vi "DragPositionScreenToPanel.vi"(8 "error in (no error)":errorcluster, 10 "DragPosition (Screen)":i32, 11 "OrderSelection in":refnum<class "OrderSelection.lvclass">) -> (0 "error out":errorcluster, 2 "DragPosition (Panel)":i32, 3 "OrderSelection out":refnum<class "OrderSelection.lvclass">)   [LabVIEW 2020, in "OrderSelection.lvclass"]
uses:
  OrderSelection.lvclass
  C:/Program Files/National Instruments/LabVIEW 2020/vi.lib/QSI/QControls/QControl Classes/GObject/GObject.lvclass
  C:/Program Files/National Instruments/LabVIEW 2020/vi.lib/QSI/QControls/QControl Classes/Generic/Generic.lvclass
  <vilib>/Utility/miscctls.llb/LVPointTypeDef.ctl
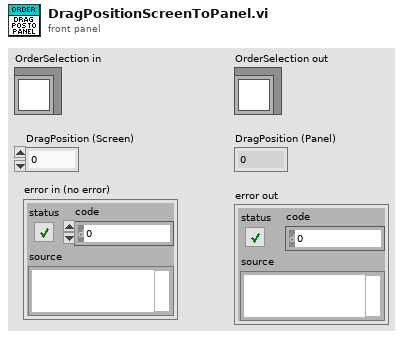
[diagram p1: front panel]
types:
  T1 = typedef "LVPointTypeDef.ctl" = cluster{"Horizontal":i16, "Vertical":i16}
  T2 = typedef "LVRectTypeDef.ctl" = cluster{"Left":i16, "Top":i16, "Right":i16, "Bottom":i16}
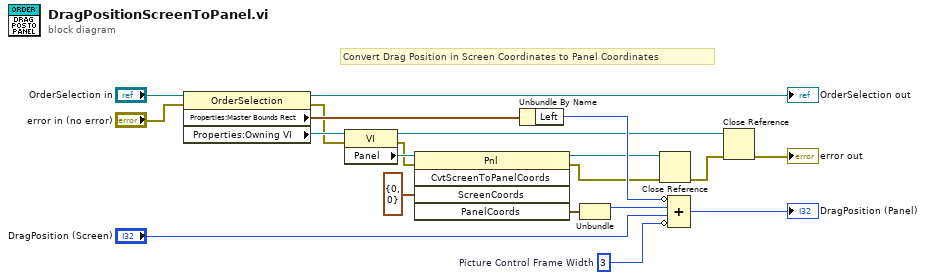
[diagram p0: block diagram]
diagram:
  w15 = 3  # Picture Control Frame Width
  # "Convert Drag Position in Screen Coordinates to Panel Coordinates"
  n1 = property class="OrderSelection"(reference="OrderSelection in", error in="error in (no error)") -> (reference out=→"OrderSelection out":refnum<class "OrderSelection.lvclass">, error out=w7:errorcluster, "Properties:Master Bounds Rect"=w14:T2, "Properties:Owning VI"=w9:refnum<vi>)
  n2 = property class="VI"(reference=w9, error in=w7) -> (reference out=w3:refnum<vi>, error out=w6:errorcluster, "Panel"=w10:refnum<vi>)
  n3 = invoke class="Pnl" method="CvtScreenToPanelCoords"(reference=w10, error in=w6, "ScreenCoords"=T1 {"Horizontal"=0, "Vertical"=0} ("Screen Coordinates")) -> (reference out=w4:refnum<vi>, error out=w5:errorcluster, "PanelCoords"=w12:T1)  [unwired: 2 in, 2 out]
  n4 = Unbundle By Name(w14) -> ("Left"=w16:i16)
  n5 = Unbundle(w12) -> ("Horizontal"=w13:i16)  [unwired: 1 out]
  n6 = Close Reference(reference=w4, error in (no error)=w5) -> (error out=w2:errorcluster)
  n7 = Compound Arithmetic op=ADD(invert w16, w13, "DragPosition (Screen)", invert w15) -> (→"DragPosition (Panel)":i32)
  n8 = Close Reference(reference=w3, error in (no error)=w2) -> (error out=→"error out":errorcluster)
